vi "sensors.vi"() -> ()   [LabVIEW 2018]
panel:
  out "Absolute_Distance (in)":dbl
  out "Distance_Along_Path":dbl
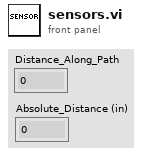
[diagram p1: front panel]
diagram:
